vi "OpenFile.vi"(8 "error in":errorcluster, 11 "路径":path) -> (0 "error out":errorcluster)   [LabVIEW 2016]
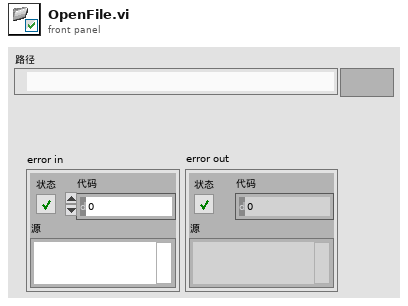
[diagram p1: front panel]
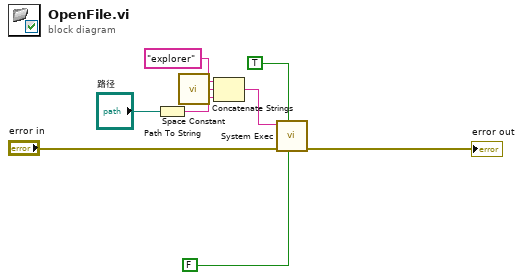
[diagram p0: block diagram]
diagram:
  n1 = Path To String(path="路径") -> (string=w5:string)
  n2 = call <vilib>:"Space Constant.vi"() -> ("String"=w7:string)
  n3 = Concatenate Strings("explorer" ("字符串"), w7, w5) -> (w9:string)
  n4 = call <vilib>:"System Exec.vi"("run minimized? (F)"=FALSE, "wait until completion? (T)"=TRUE, "error in (no error)"="error in", "command line"=w9) -> ("error out"=→"error out":errorcluster)  [unwired: 4 in, 3 out]
